vi "libssh2_agent_get_identity_path.vi"(8 "error in (no error)":errorcluster, 11 "agent":T1) -> (0 "error out":errorcluster, 2 "path":path)   [LabVIEW 2013, in "libssh2.lvlib"]
doc: "Get the path to the identity socket previously set with <B>libssh2_agent_set_identity_path</B>."
uses:
  libssh2.lvlib
  Agent Refnum.ctl
  Acquire Session.vi
  Release Session.vi
  Not An Agent.vi
  <vilib>/Utility/error.llb/Error Cluster From Error Code.vi
  Global Settings.vi
  Read Agent Refnum.vi
  Read Session Refnum.vi
  <vilib>/Utility/semaphor.llb/Acquire Semaphore.vi
  <vilib>/Utility/semaphor.llb/Release Semaphore.vi
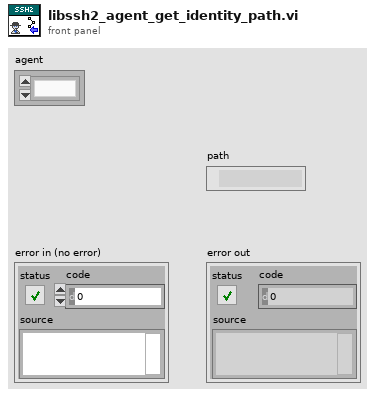
[diagram p1: front panel]
types:
  T1 = typedef "libssh2.lvlib/Agent Refnum.ctl" = refnum<k1>
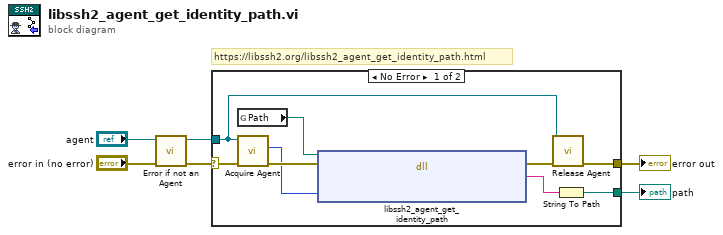
[diagram p0: block diagram]
diagram:
  # "https://libssh2.org/libssh2_agent_get_identity_path.html"
  n1 = call "Error if not an Agent.vi"("error in (no error)"="error in (no error)", "agent"="agent") -> ("error out"=w3:errorcluster, "agent out"=w2:T1)  [unwired: 8 in]
  n2 = case shown="No Error" w3 {
    selector: w3 -> [w14 w16]
    tunnel: [w8 w16] -> w6
    tunnel: w2 -> [w7 _]
    tunnel: [w13 _] -> w4
    frame No Error {
      n3 = global read "Global Settings.vi" "Path"() -> (w12:path)
      n4 = call "Acquire Agent.vi"("error in (no error)"=w14, "agent"=w7) -> ("error out"=w11:errorcluster, "LIBSSH2_AGENT*"=w10:u64)  [unwired: 8 in]
      n5 = dll-call lib="?" fn="libssh2_agent_get_identity_path"(path in=w12, error in=w11, "agent"=w10) -> (error out=w15:errorcluster, "return value"=w9:string)  [unwired: 2 in, 1 out]
      n6 = call "Release Agent.vi"("error in (no error)"=w15, "agent"=w7) -> ("error out"=w8:errorcluster)  [unwired: 9 in]
      n7 = String To Path(string=w9) -> (path=w13:path)
    }
    frame Error {
    }
  }
  "error out" <- w6
  "path" <- w4
